vi "Peg-in-hole 2015-03-02 data.vi"() -> ()   [LabVIEW 2013]
uses:
  <vilib>/Analysis/baseanly.llb/Mean (DBL).vi
  <vilib>/Analysis/NI_AALBase.lvlib
panel:
  out "XY Graph":cluster{cluster{dbl, "mean":dbl}[]}[](graph)
  in  "2015-03-02":dbl[](array[numeric])=[27.75, 28.05, 27.9, 17.75, 143.25, 110.6, 42.95, 17.2, 41.6, 16.8, 27.95, 65.9, 30.25, 18.5, 17.5, 48.1, 62.35, 17.55, 52.75, 322.0, 27.9, 27.45, 27.2, 18.0, 17.4, 27.95, 51.2, 17.55, 40.2, 171.4, 28.25, 27.85, 27.35, 17.85, 16.95, 39.3, 38.75, 17.35, 29.45, 17.2, 27.8, 28.15, 142.2, 63.6, 17.65, 89.651, 28.5, 17.55, 29.0, 17.15, 17.65, 28.45, 28.45, 42.9, 16.75, 38.55, 39.45, 17.8, 208.85, 49.9, 17.25, 37.75, 69.85, 29.9, 17.3, 17.5, 19.1, 80.35, 31.499, 80.55, 17.45, 17.65, 27.95, 40.65, 17.25, 70.15, 28.8, 17.4, 18.4, 17.55, 16.95, 50.4, 27.15, 52.5, 16.85, 17.6, 39.6, 17.35, 18.35, 17.75, 58.15, 71.55, 27.65, 107.75, 16.95, 28.75, 28.7, 17.5, 128.9, 59.35]
  # "single taught point"
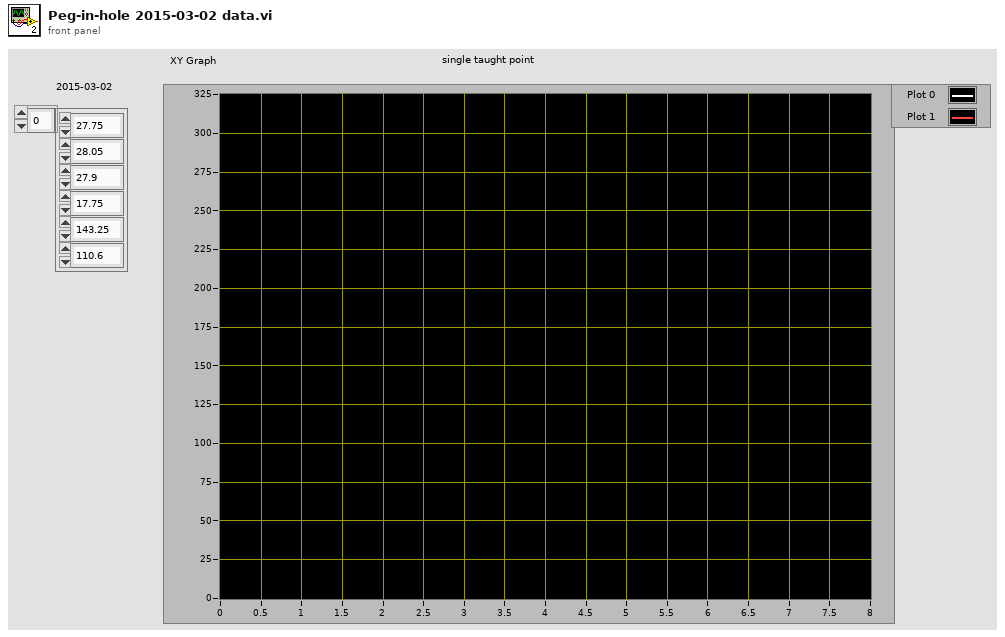
[diagram p1: front panel]
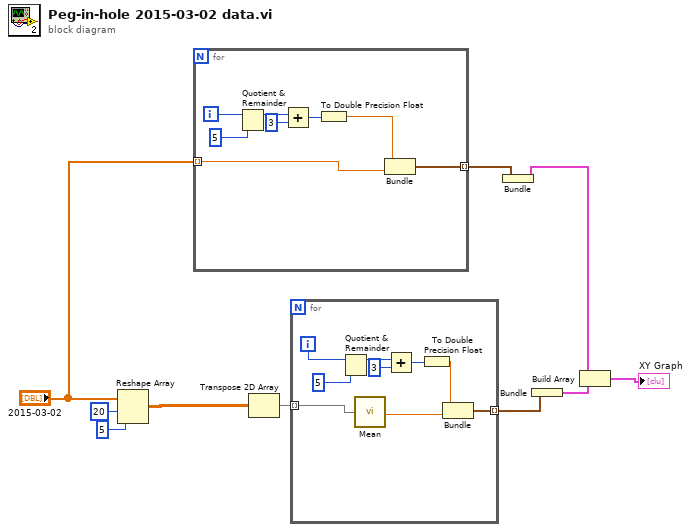
[diagram p0: block diagram]
diagram:
  n1 = Reshape Array("2015-03-02", 20 ("dimension size"), 5 ("dimension size")) -> (w8:dbl[][])
  n2 = for {
    tunnel: "2015-03-02" -> [w12] mode=indexing
    tunnel: [w11] -> w5 mode=indexing
    i -> [w18]
    n3 = Quotient & Remainder(x=w18, y=5) -> (x-y*floor(x/y)=w16:i32)  [unwired: 1 out]
    n4 = Add(x=w16, y=3) -> (x+y=w14:i32)
    n5 = To Double Precision Float(number=w14) -> (double precision float=w13:dbl)
    n6 = Bundle(w13, w12) -> (w11:cluster{dbl, dbl})  [unwired: 1 in]
  }
  n7 = Transpose 2D Array(2D array=w8) -> (transposed array=w7:dbl[][])
  n8 = for {
    tunnel: w7 -> [w27] mode=indexing
    tunnel: [w19] -> w3 mode=indexing
    i -> [w22]
    n9 = Quotient & Remainder(x=w22, y=5) -> (x-y*floor(x/y)=w25:i32)  [unwired: 1 out]
    n10 = call-poly <vilib>:"Mean.vi"("X"=w27) -> ("mean"=w20:dbl)  [unwired: 1 out]
    n11 = Add(x=w25, y=3) -> (x+y=w23:i32)
    n12 = To Double Precision Float(number=w23) -> (double precision float=w21:dbl)
    n13 = Bundle(w21, "mean"=w20) -> (w19:cluster{dbl, "mean":dbl})  [unwired: 1 in]
  }
  n14 = Bundle(w5) -> (w6:cluster{cluster{dbl, dbl}[]})  [unwired: 1 in]
  n15 = Bundle(w3) -> (w4:cluster{cluster{dbl, "mean":dbl}[]})  [unwired: 1 in]
  n16 = Build Array(w6, w4) -> (→"XY Graph":cluster{cluster{dbl, "mean":dbl}[]}[])
